vi "LastScanPassedGreen.vi"(8 "error in (no error)":errorcluster, 9 "Next Tray Cnt":u32, 10 "Trays":u32, 11 "Tray":u32) -> (0 "error out":errorcluster)   [LabVIEW 2013]
panel:
  out "String":string
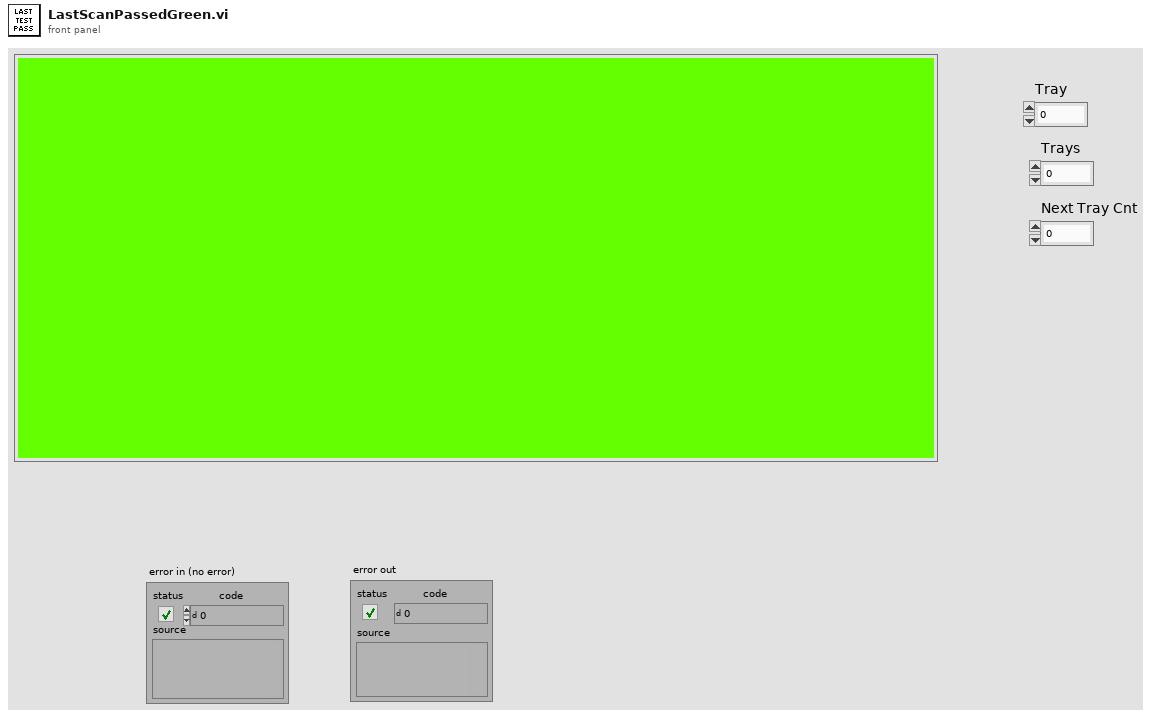
[diagram p1: front panel]
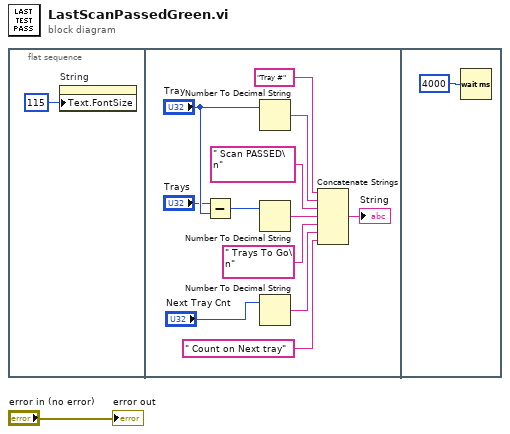
[diagram p0: block diagram]
diagram:
  n1 = flat-sequence {
    frame #0 {
      n2 = property on="String" class="Str"("Text.FontSize"=u32 115 ("Text.Font:Size")) -> ()  [unwired: 2 in, 2 out]
    }
    frame #1 {
      n3 = Subtract(x="Trays", y="Tray") -> (x-y=w12:u32)
      n4 = Number To Decimal String(number="Tray") -> (decimal integer string=w7:string)  [unwired: 1 in]
      n5 = Number To Decimal String(number=w12) -> (decimal integer string=w13:string)  [unwired: 1 in]
      n6 = Number To Decimal String(number="Next Tray Cnt") -> (decimal integer string=w4:string)  [unwired: 1 in]
      n7 = Concatenate Strings("Tray #" ("string"), w7, " Scan PASSED\n" ("string"), w13, " Trays To Go\n" ("string"), w4, " Count on Next tray" ("string")) -> (→"String":string)
    }
    frame #2 {
      n8 = Wait (ms)(milliseconds to wait=u32 4000) -> ()  [unwired: 1 out]
    }
  }
  "error out" <- "error in (no error)"
